vi "Check ID for Message.vi"(7 "ID":string, 8 "error in (no error)":errorcluster, 11 "Major Frame in":refnum<class "Major Frame.lvclass">) -> (0 "error out":errorcluster, 2 "Msg Found?":bool, 3 "Major Frame out":refnum<class "Major Frame.lvclass">, 5 "Message":refnum<class "Message.lvclass">)   [LabVIEW 2020, in "BCI-1553 API.lvlib" / "Major Frame.lvclass"]
doc: "Verifies if an ID corresponds to a message."
uses:
  Major Frame.lvclass
  Message/Message.lvclass
  Major Frame.lvclass/Major Frame.ctl
  Dependencies/Registry/Registry.lvclass/Registry.ctl
  Dependencies/Registry/Registry.lvclass
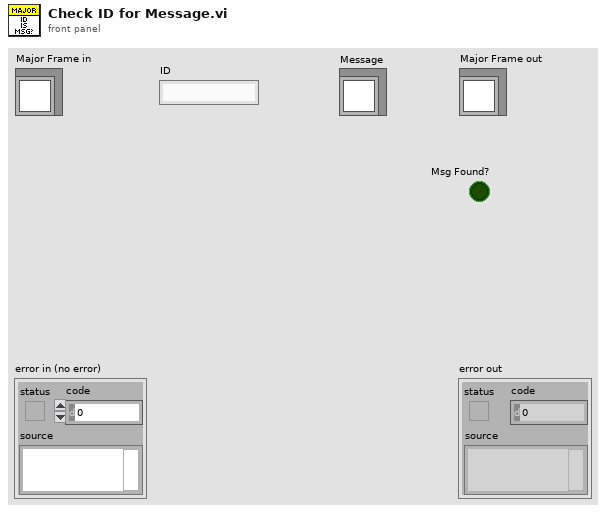
[diagram p1: front panel]
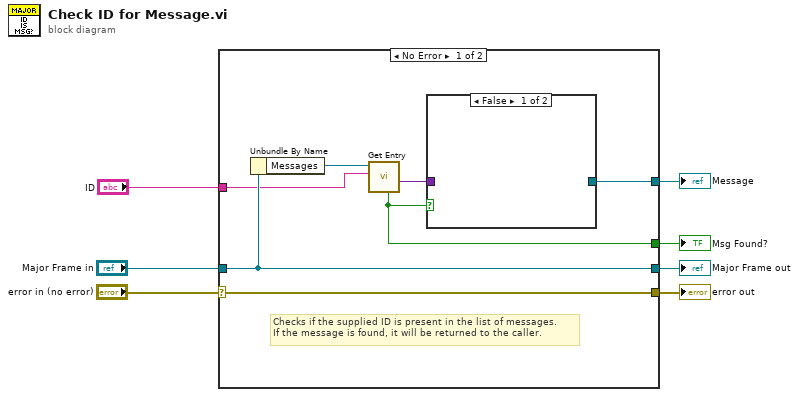
[diagram p0: block diagram]
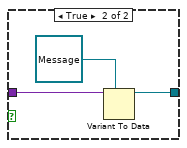
[diagram p2: hidden frame]
diagram:
  n1 = case shown="No Error" "error in (no error)" {
    selector: "error in (no error)" -> [w14 w19]
    tunnel: [w14 w19] -> w6
    tunnel: [w13 w18] -> w4
    tunnel: "Major Frame in" -> [w13 w18]
    tunnel: "ID" -> [w11 _]
    tunnel: [w9 _] -> w2
    tunnel: [w8 _] -> w1
    frame No Error {
      # "Checks if the supplied ID is present in the list of messages.\nIf the message is found, it will be returned to the caller."
      n2 = Unbundle By Name(w13) -> ("Messages"=w12:refnum<class "Registry.lvclass">)
      n3 = call "Get Entry.vi"("Key"=w11, "Registry in"=w12) -> ("Value"=w10:variant, "Found?"=w9:bool)  [unwired: 6 in, 2 out]
      n4 = case shown="False" w9 {
        tunnel: w10 -> [_ w17]
        tunnel: [_ w15] -> w8
        frame False {
        }
        frame True {
          n5 = Variant To Data(type=refnum<class "Message.lvclass"> refnum ("Message"), Variant=w17) -> (data=w15:refnum<class "Message.lvclass">)  [unwired: 1 in, 1 out]
        }
      }
    }
    frame Error {
    }
  }
  "error out" <- w6
  "Major Frame out" <- w4
  "Message" <- w1
  "Msg Found?" <- w2
